vi "App - FileSync.vi"(8 "error in (no error)":errorcluster) -> (0 "error out":errorcluster)   [LabVIEW 2020]
uses:
  FTP/FTPProtocol/FTPProtocol.lvclass
  C:/Users/yaoli/Desktop/FileSync/Base/Protocol/Protocol.lvclass
  Base/FileSync -- Base.lvlib
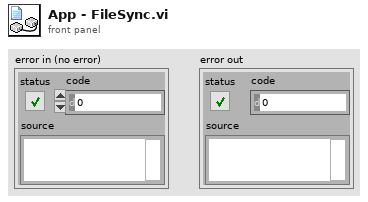
[diagram p1: front panel]
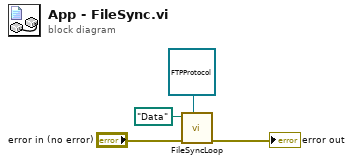
[diagram p0: block diagram]
diagram:
  n1 = call "FileSyncLoop.vi"("Protocol.lvclass"=refnum<class "FTPProtocol.lvclass"> refnum ("FTPProtocol"), "error in"="error in (no error)", "Path"=path "Data") -> ("error out"=→"error out":errorcluster)  [unwired: 8 in]
